vi "healLV.vi"() -> ()   [LabVIEW 2020]
panel:
  out "SpO2":dbl(knob) scale=0.0..100.0
  out "Heart Rate":dbl(knob) scale=0.0..200.0
  out "SpO2":dbl
  in  "?":bool
  out "Heart Rate Waveform":dbl(graph)
  out "Heart Rate":dbl
  in  "IP Adress":string
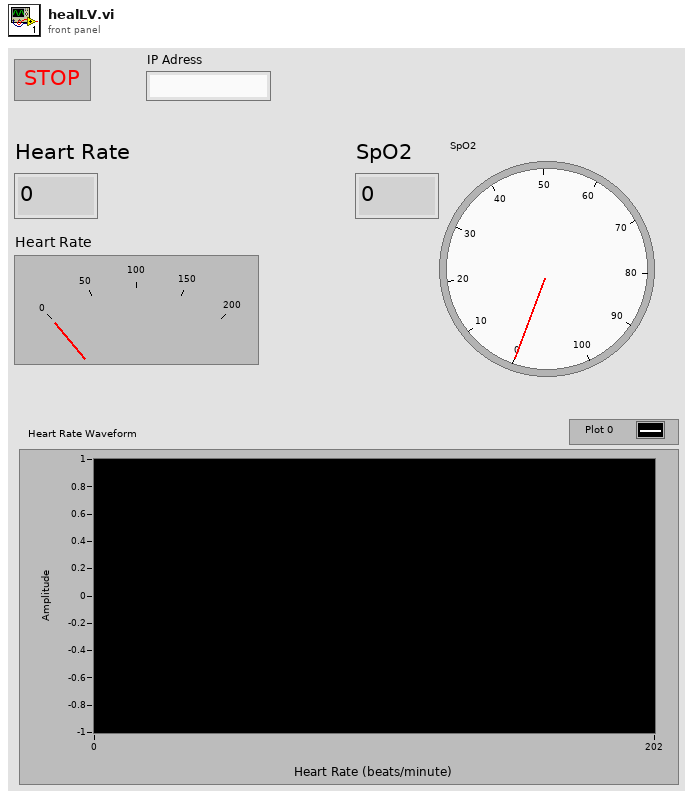
[diagram p1: front panel]
types:
  T1 = enum16{"Standard", "Buffered", "CRLF", "Immediate"}
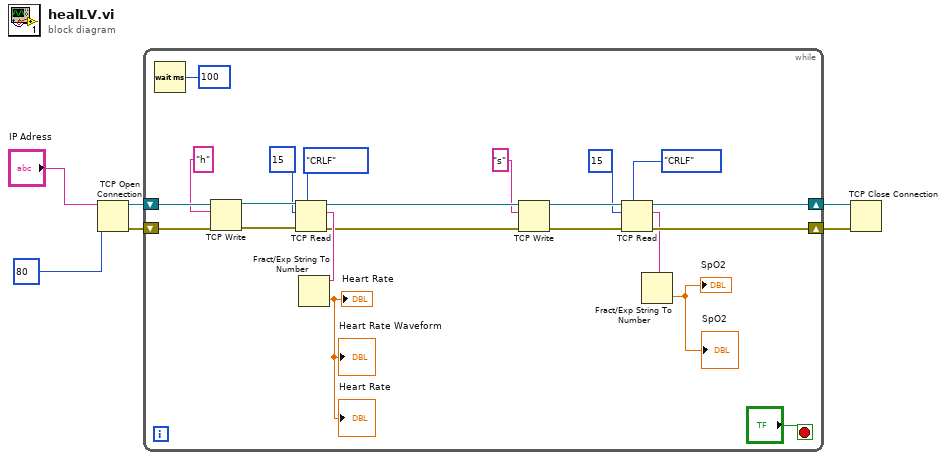
[diagram p0: block diagram]
diagram:
  n1 = TCP Open Connection(address="IP Adress", remote port or service name=u16 80) -> (connection ID=w4:refnum<k5>, error out=w2:errorcluster)  [unwired: 3 in]
  n2 = while {
    shift-right: [w17] -> w3
    shift-left: w4 -> [w28]
    shift-right: [w11] -> w1
    shift-left: w2 -> [w26]
    stop <- "?" stop-if-true
    n3 = Wait (ms)(milliseconds to wait=u32 100) -> ()  [unwired: 1 out]
    n4 = TCP Write(connection ID=w28, data in="h", error in (no error)=w26) -> (connection ID out=w27:refnum<k5>, error out=w25:errorcluster)  [unwired: 1 in, 1 out]
    n5 = TCP Read(connection ID=w27, bytes to read=15, error in (no error)=w25, 7:T1."CRLF" ("mode (standard)")) -> (connection ID out=w19:refnum<k5>, data out=w21:string, error out=w16:errorcluster)  [unwired: 1 in]
    n6 = Fract/Exp String To Number(string=w21) -> (number=→"Heart Rate" →"Heart Rate Waveform" →"Heart Rate":dbl)  [unwired: 3 in, 1 out]
    n7 = TCP Write(connection ID=w19, data in="s", error in (no error)=w16) -> (connection ID out=w18:refnum<k5>, error out=w15:errorcluster)  [unwired: 1 in, 1 out]
    n8 = TCP Read(connection ID=w18, bytes to read=15, error in (no error)=w15, 7:T1."CRLF" ("mode (standard)")) -> (connection ID out=w17:refnum<k5>, data out=w10:string, error out=w11:errorcluster)  [unwired: 1 in]
    n9 = Fract/Exp String To Number(string=w10) -> (number=→"SpO2" →"SpO2":dbl)  [unwired: 3 in, 1 out]
  }
  n10 = TCP Close Connection(connection ID=w3, error in (no error)=w1) -> ()  [unwired: 1 in, 2 out]
